vi "Remove Special Chars.vi"(9 "String in":string) -> (3 "String out":string)   [LabVIEW 2018]
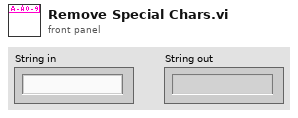
[diagram p1: front panel]
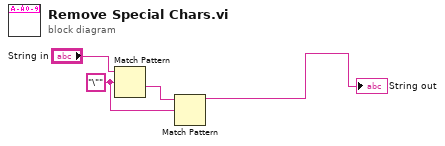
[diagram p0: block diagram]
diagram:
  w3 = "\"" ("regular expression")
  n1 = Match Pattern(string="String in", regular expression=w3) -> (after substring=w4:string)  [unwired: 1 in, 3 out]
  n2 = Match Pattern(string=w4, regular expression=w3) -> (before substring=→"String out":string)  [unwired: 1 in, 3 out]
